vi "GeraGrafico.vi"(0 "quant":dbl, 1 "Tensao in":dbl[](array[numeric]), 5 "appended path":path, 9 "size":i32, 11 "notificacao rapida - in":string, 12 "counts in":dbl[](array[numeric])) -> (3 "notificacao rapida -out":string, 4 "Tensao out":dbl[](array[numeric]), 6 "Table Control":string[][](table), 8 "error":bool, 10 "RUN":dbl, 14 "XY Graph":cluster{"X":dbl[], "Y":dbl[]}[](array[cluster]), 15 "counts out":dbl[](array[numeric]))   [LabVIEW 2018]
panel:
  out "Texto Geral":string="\r"
  in  "discrepancia":bool
  in  "discrepancia":string
  in  "texto-geral":string
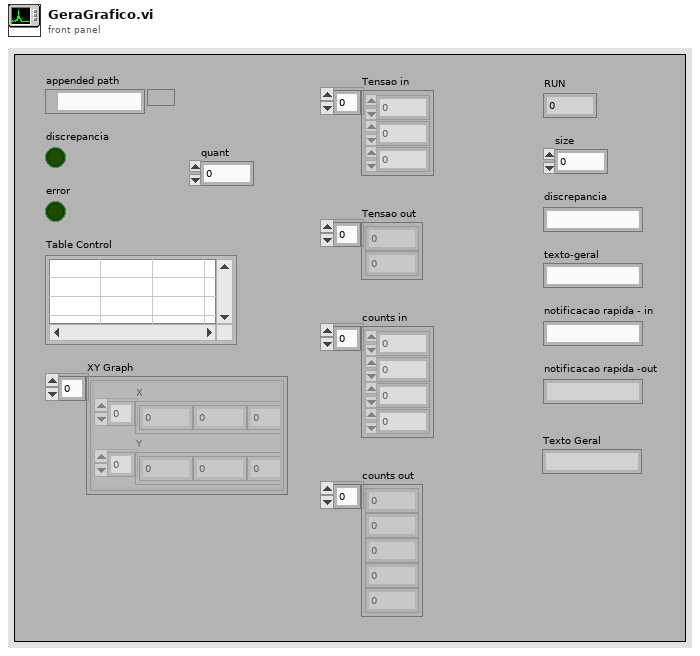
[diagram p1: front panel]
types:
  T1 = enum16{"open", "replace", "create", "open or create", "replace or create", "replace or create with confirmation"}
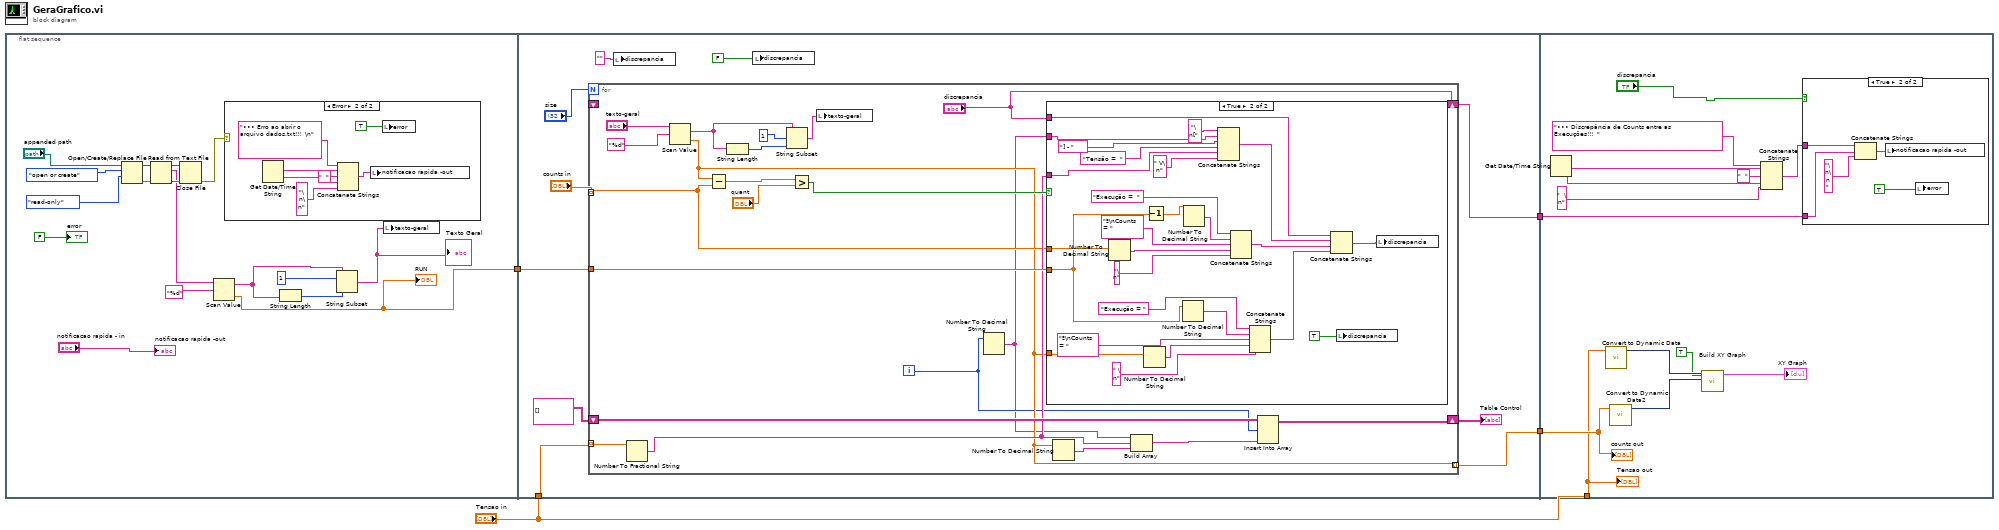
[diagram p0: block diagram]
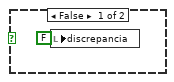
[diagram p4: hidden frame]
diagram:
  n1 = flat-sequence {
    tunnel: [w7] -> w3
    tunnel: [w32] -> w4
    tunnel: "Tensao in" -> [w37]
    tunnel: w3 -> [w31]
    tunnel: [w29] -> w1
    tunnel: "Tensao in" -> [w94]
    tunnel: w4 -> [w87]
    tunnel: w1 -> [w96]
    frame #0 {
      n2 = Open/Create/Replace File(file path (use dialog)="appended path", operation (0:open)=T1."open or create", access (0:read/write)=enum16{"read/write", "read-only", "write-only"}."read-only") -> (refnum out=w18:refnum<file>, error out=w20:errorcluster)  [unwired: 3 in, 1 out]
      n3 = Read from Text File(file (use dialog)=w18, error in=w20) -> (refnum out=w17:refnum<file>, text=w15:string, error out=w16:errorcluster)  [unwired: 2 in, 1 out]
      n4 = Close File(refnum=w17, error in=w16) -> (error out=w10:errorcluster)  [unwired: 1 out]
      n5 = Scan Value(string=w15, format string="%d") -> (output string=w11:string, value=w7:dbl)  [unwired: 1 in]
      "RUN" <- w7
      n6 = case shown="Error" w10 {
        frame No Error {
        }
        frame Error {
          n7 = Get Date/Time String() -> (date string=w26:string, time string=w23:string)  [unwired: 3 in]
          n8 = Concatenate Strings("••• Erro ao abrir o arquivo dados.txt!!!  \n", w26, "  " ("string"), w23, "\n\n" ("string")) -> (w25:string)
          n9 = local write "notificacao rapida -out"(w25) -> ()
          n10 = local write "error"(TRUE ("Boolean 2")) -> ()
        }
      }
      n11 = String Length(string=w11) -> (length=w13:i32)
      n12 = String Subset(string=w11, offset (0)=1, length (rest)=w13) -> (substring=w5:string)
      "Texto Geral" <- w5
      n13 = local write "texto-geral"(w5) -> ()
      "error" <- FALSE ("Boolean 2")
      "notificacao rapida -out" <- "notificacao rapida - in"
    }
    frame #1 {
      n14 = for {
        N: "size" -> [_]
        tunnel: "counts in" -> [w43] mode=indexing
        shift-right: ["discrepancia"] -> w32
        shift-left: _ -> [_]
        tunnel: w37 -> [w54] mode=indexing
        tunnel: w31 -> [w52]
        shift-right: [w48] -> w30
        shift-left: string[][] [] ("Table Control") -> [w50]
        tunnel: [w41] -> w29 mode=indexing
        i -> [w40]
        n15 = Number To Fractional String(number=w54) -> (F-format string=w47:string)  [unwired: 3 in]
        n16 = Scan Value(string="texto-geral", format string="%d") -> (output string=w58:string, value=w41:dbl)  [unwired: 1 in]
        n17 = Subtract(x=w41, y=w43) -> (x-y=w42:dbl)
        n18 = String Length(string=w58) -> (length=w57:i32)
        n19 = String Subset(string=w58, offset (0)=1, length (rest)=w57) -> (substring=w49:string)
        n20 = Greater?(x=w42, y="quant") -> (0:w55:bool)
        n21 = local write "texto-geral"(w49) -> ()
        n22 = Number To Decimal String(number=w40) -> (decimal integer string=w39:string)  [unwired: 1 in]
        n23 = case shown="True" w55 {
          tunnel: "discrepancia" -> [_ w81]
          tunnel: w52 -> [_ w78]
          tunnel: w43 -> [_ w79]
          tunnel: w41 -> [_ w77]
          tunnel: w47 -> [_ w76]
          tunnel: w39 -> [_ w61]
          frame False {
          }
          frame True {
            n24 = Number To Decimal String(number=w79) -> (decimal integer string=w73:string)  [unwired: 1 in]
            n25 = Number To Decimal String(number=w77) -> (decimal integer string=w70:string)  [unwired: 1 in]
            n26 = Decrement(x=w78) -> (x-1=w80:dbl)
            n27 = Number To Decimal String(number=w78) -> (decimal integer string=w64:string)  [unwired: 1 in]
            n28 = Number To Decimal String(number=w80) -> (decimal integer string=w67:string)  [unwired: 1 in]
            n29 = Concatenate Strings("\n[" ("string"), w61, "] - " ("string"), "Tensão =  " ("string"), w76, " V\n" ("string")) -> (w75:string)
            n30 = Concatenate Strings("Execução =  " ("string"), w67, "º\nCounts = " ("string"), w73, "\n" ("string")) -> (w66:string)
            n31 = Concatenate Strings("Execução = " ("string"), w64, "º\nCounts = " ("string"), w70, " \n" ("string")) -> (w63:string)
            n32 = Concatenate Strings(w81, w75, w66, w63) -> (w83:string)
            n33 = local write "discrepancia"(TRUE ("Boolean")) -> ()
            n34 = local write "discrepancia"(w83) -> ()
          }
        }
        n35 = Number To Decimal String(number=w41) -> (decimal integer string=w46:string)  [unwired: 1 in]
        n36 = Build Array(w39, w47, w46) -> (w51:string[])
        n37 = Insert Into Array(array=w50, index (row)=w40, new element=w51) -> (w48:string[][])  [unwired: 1 in]
      }
      "Table Control" <- w30
      n38 = local write "discrepancia"("" ("String")) -> ()
      n39 = local write "discrepancia"(FALSE ("Boolean")) -> ()
    }
    frame #2 {
      n40 = Get Date/Time String() -> (date string=w92:string, time string=w89:string)  [unwired: 3 in]
      n41 = call "Convert to Dynamic Data"("Array"=w94) -> ("Dynamic Data Type"=w99:dynamicdata)  [unwired: 3 in]
      n42 = call "Convert to Dynamic Data2"("Array"=w96) -> ("Dynamic Data Type"=w97:dynamicdata)  [unwired: 3 in]
      n43 = call "Build XY Graph"("Enable"=TRUE, "Y Input"=w97, "X Input"=w99) -> ("XY Graph"=→"XY Graph":cluster{"X":dbl[], "Y":dbl[]}[])  [unwired: 7 in, 1 out]
      n44 = Concatenate Strings("••• Discrepância de Counts entre as Execuções!!!  ", w92, "  " ("string"), w89, "  \n" ("string")) -> (w91:string)
      n45 = case shown="True" "discrepancia" {
        tunnel: w87 -> [_ w105]
        tunnel: w91 -> [_ w101]
        frame False {
          n46 = local write "discrepancia"(FALSE ("Boolean")) -> ()
        }
        frame True {
          n47 = Concatenate Strings(w101, w105, "\n\n " ("string")) -> (w104:string)
          n48 = local write "notificacao rapida -out"(w104) -> ()
          n49 = local write "error"(TRUE ("Boolean 2")) -> ()
        }
      }
      "counts out" <- w96
      "Tensao out" <- w94
    }
  }
